vi "Polls.Compile.vi"(8 "error in (no error)":errorcluster, 11 "Section Ref in":T6 format="%.0x") -> (0 "error out":errorcluster, 1 "Poll Settings":T1[](array[typedef]), 2 "Service Channels":T3[](array[typedef]) {"Signal.Cmd.Refs"."Signal Refs" format="%.0x"; "Signal.Cmd.Info"."Signals"."Byte Order" items=["Little Endian", "Big Endian"]; "Signal.Cmd.Info"."Signals"."Data Type" items=["Signed", "Unsigned", "IEEE Float"]; "Settings.Refs"."Signal Refs" format="%.0x"; "Signal.Resp.Refs"."Signal Refs" format="%.0x"; "Signal.Resp.Info"."Signals"."Byte Order" items=["Little Endian", "Big Endian"]; "Signal.Resp.Info"."Signals"."Data Type" items=["Signed", "Unsigned", "IEEE Float"]; "Trigger.Refs"."Signal Refs" format="%.0x"; "Status.Refs"."Signal Refs" format="%.0x"}, 3 "Section Ref out":T6 format="%.0x")   [LabVIEW 2019, in "Diagnostics Addon System Explorer.lvlib"]
uses:
  Diagnostics Addon System Explorer.lvlib
  <vilib>/NI VeriStand/Custom Device API/Custom Device Item Ref.ctl
  Types/Service.Export.ctl
  Types/Frame.Ref.ctl
  Addon Shared/Types/Type.ctl
  Addon Shared/Types/Frame.Compile.ctl
  Addon Shared/Types/Signal.ctl
  Addon Shared/Types/Poll.Compiled.ctl
  Addon Shared/Types/DPID.Rate.ctl
  Types/FG.Action.ctl
  Addon Shared/SubVIs/Constants.vi
  <vilib>/NI VeriStand/Custom Device Tools/Custom Device Utility Library/NI VeriStand - Search for All Items by GUID.vi
  <vilib>/NI VeriStand/Custom Device Tools/Custom Device Utility Library/NI VeriStand - Search for Item by GUID.vi
  <vilib>/NI VeriStand/Custom Device API/NI VeriStand - Get Item Children.vi
  <vilib>/NI VeriStand/Custom Device Tools/Custom Device Utility Library/NI VeriStand - Search for Item by Name.vi
  <vilib>/NI/NI VeriStand Advanced SysDef API/SysDef API/SysDef.Property.Set.vi
  <vilib>/NI/NI VeriStand Advanced SysDef API/_SubVIs/SysDef.Property.Set.U32.vi
  <vilib>/NI VeriStand/Custom Device API/NI VeriStand - Get Item Property.vi
  <vilib>/NI VeriStand/Custom Device API/Get Item Property (U32).vi
  <vilib>/NI VeriStand/Custom Device Tools/Custom Device Utility Library/Custom Device Utility Library.lvlib
  <vilib>/NI VeriStand/Custom Device API/Custom Device API.lvlib
  Addon Shared/Diagnostics Addon Shared.lvlib
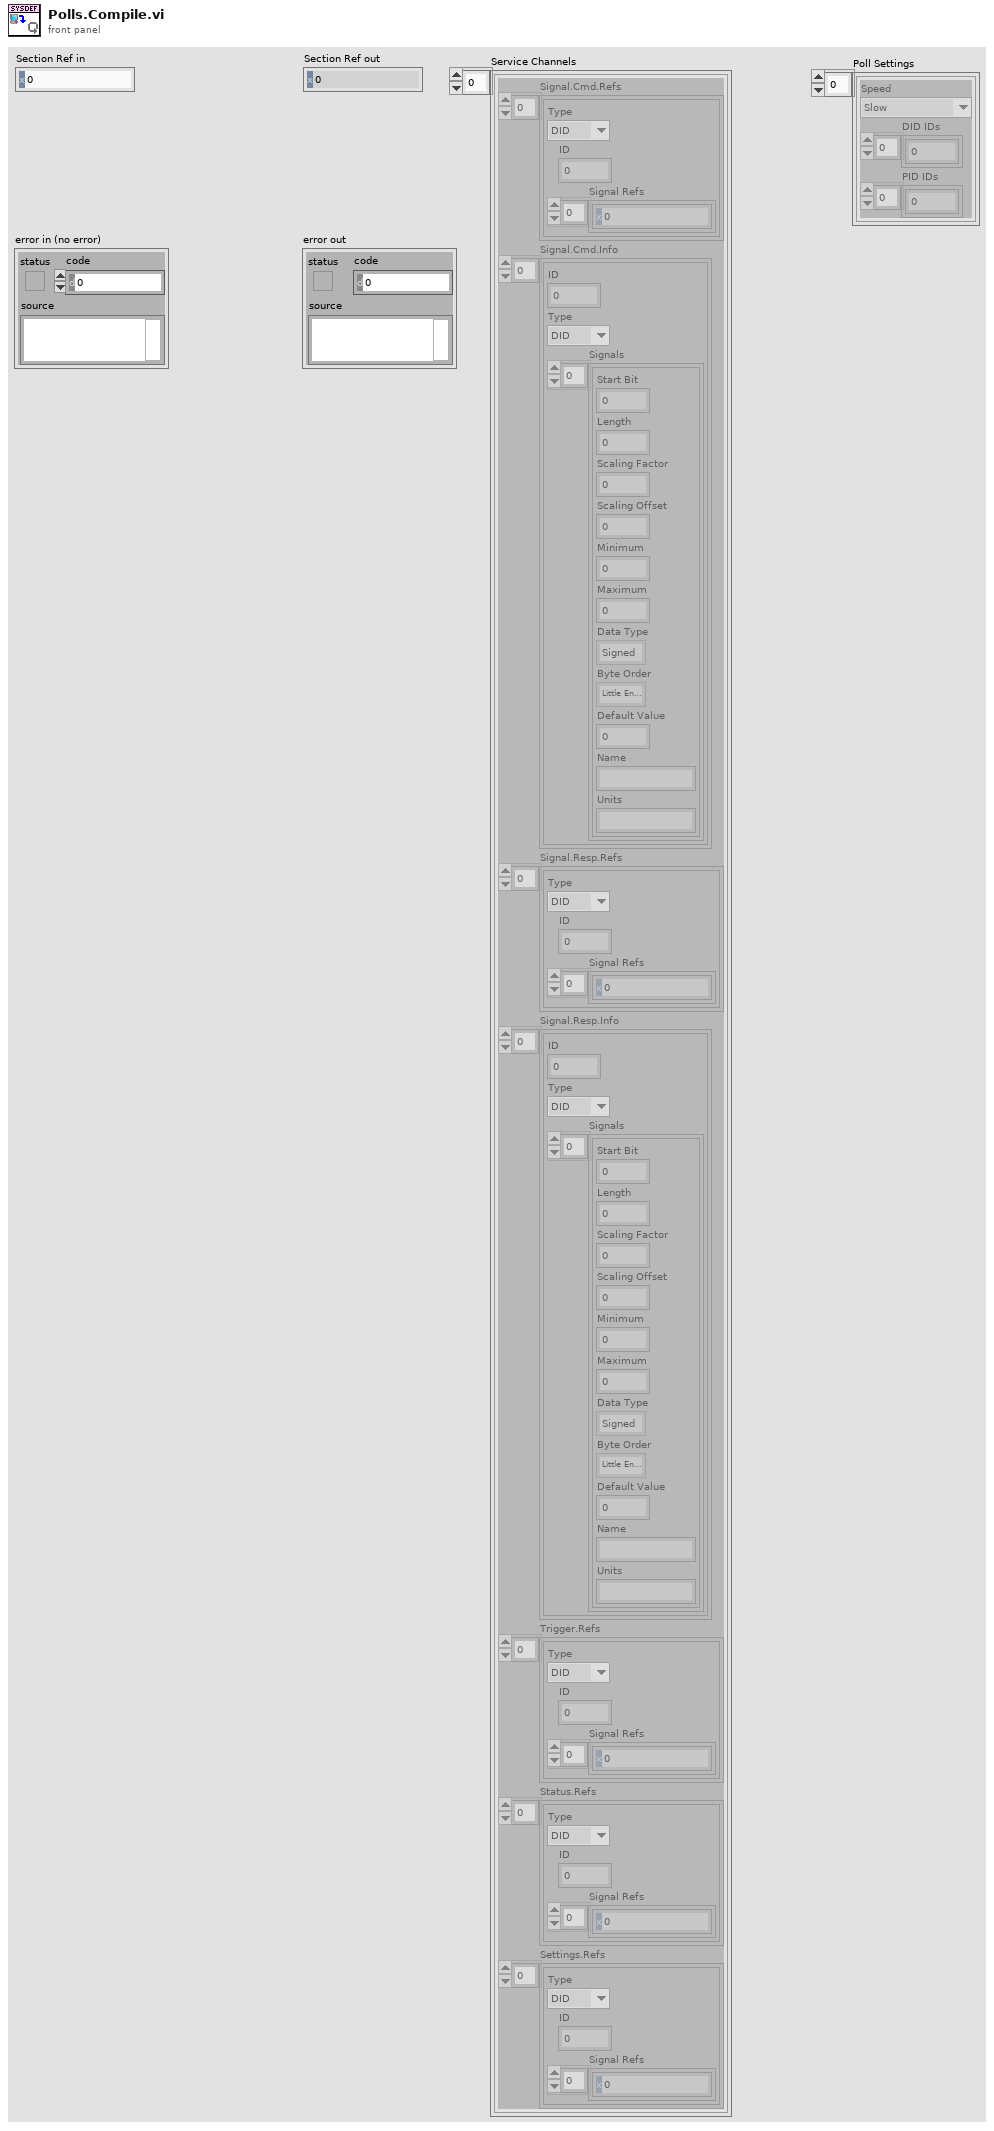
[diagram p1: front panel]
types:
  T1 = typedef "Diagnostics Addon Shared.lvlib/Poll.Compiled.ctl" = cluster{"Speed":T2, "DID IDs":u32[], "PID IDs":u32[]}
  T2 = typedef "Diagnostics Addon Shared.lvlib/DPID.Rate.ctl" = enum16{"Slow", "Medium", "Fast"}
  T3 = typedef "Diagnostics Addon System Explorer.lvlib/Service.Export.ctl" = cluster{"Signal.Cmd.Refs":T4[], "Signal.Cmd.Info":T7[], "Signal.Resp.Refs":T4[], "Signal.Resp.Info":T7[], "Trigger.Refs":T4[], "Status.Refs":T4[], "Settings.Refs":T4[]}
  T4 = typedef "Diagnostics Addon System Explorer.lvlib/Frame.Ref.ctl" = cluster{"Type":T5, "ID":u32, "Signal Refs":T6[]}
  T5 = typedef "Diagnostics Addon Shared.lvlib/Type.ctl" = enum16{"DID", "CDID", "PID", "CPID", "Read Memory", "Write Memory", "IO Control", "Routine Start", "Routine Request", "Routine Stop", "User Defined", "DTC Control", "Clear DTCs", "Read DTCs", "Start DTCs", "DTC Change Count", "Tester Present", "Unlock ECU", "Reset ECU", "Diag Session Control", "Communication Control", "DPID Control", "Poll Control", "Diag CAN Control"}
  T6 = typedef "Custom Device API.lvlib/Custom Device Item Ref.ctl" = u64
  T7 = typedef "Diagnostics Addon Shared.lvlib/Frame.Compile.ctl" = cluster{"ID":u32, "Type":T5, "Signals":T8[]}
  T8 = typedef "Diagnostics Addon Shared.lvlib/Signal.ctl" = cluster{"Start Bit":u32, "Length":u32, "Scaling Factor":dbl, "Scaling Offset":dbl, "Minimum":dbl, "Maximum":dbl, "Data Type":u32, "Byte Order":u32, "Default Value":dbl, "Name":string, "Units":string}
  T9 = typedef "Diagnostics Addon System Explorer.lvlib/FG.Action.ctl" = enum16{"Get", "Set"}
  T10 = typedef "Diagnostics Addon System Explorer.lvlib/Poll.Settings.ctl" = cluster{"Input Channels":T11[], "Speed":T2}
  T11 = typedef "Diagnostics Addon System Explorer.lvlib/Poll.LinkedNode.ctl" = cluster{"Node ID":u64}
  T12 = typedef "Custom Device API.lvlib/Custom Device Item Info.ctl" = cluster{"Name":string, "Is Channel":bool, "GUID":string, "Is Waveform":bool}
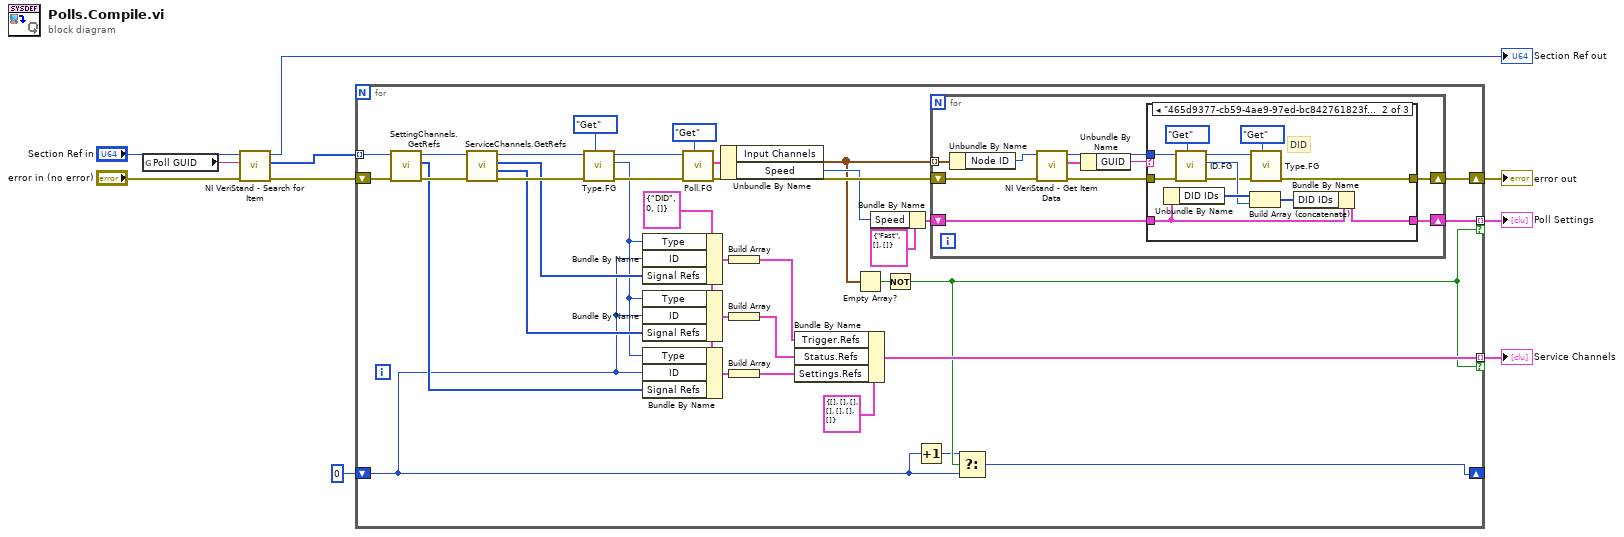
[diagram p0: block diagram]
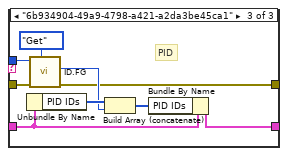
[diagram p3: hidden frame]
diagram:
  n1 = global read "Constants.vi" "Poll GUID"() -> (w10:string)
  n2 = call-poly <vilib>:"NI VeriStand - Search for Item.vi"("error in"="error in (no error)", "Item GUID"=w10, "Section Ref in"="Section Ref in") -> ("error out"=w9:errorcluster, "Item Refs"=w8:T6[], "Section Ref out"=→"Section Ref out":T6)  [unwired: 5 in, 1 out]
  n3 = for {
    tunnel: w8 -> [w15] mode=indexing
    shift-right: [w40] -> w5
    shift-left: w9 -> [w38]
    tunnel: [w41] -> w2 mode=indexing if=w14
    tunnel: [w17] -> w3 mode=indexing if=w14
    shift-right: [w13] -> _
    shift-left: 0 -> [w11]
    w27 = T4 {"Type"=enum."DID", "ID"=0, "Signal Refs"=[]} ("cluster")
    n4 = call "SettingChannels.GetRefs.vi"("error in (no error)"=w38, "Item Ref in"=w15) -> ("error out"=w34:errorcluster, "Settings"=w24:T6[], "Section Ref out"=w33:T6)  [unwired: 7 in]
    n5 = call "ServiceChannels.GetRefs.vi"("error in (no error)"=w34, "Item Ref in"=w33) -> ("error out"=w32:errorcluster, "Status"=w25:T6[], "Trigger"=w26:T6[], "Section Ref out"=w31:T6)  [unwired: 6 in]
    n6 = call "Type.FG.vi"("Action"=FG.Action."Get", "error in (no error)"=w32, "Device Item Ref in"=w31) -> ("error out"=w37:errorcluster, "Type"=w20:T5, "Device Item Ref out"=w16:T6)  [unwired: 6 in]
    n7 = Bundle By Name(cluster=w27, "Type"=w20, "ID"=w11, "Signal Refs"=w26) -> (w30:T4)
    n8 = Bundle By Name(cluster=w27, "Type"=w20, "ID"=w11, "Signal Refs"=w25) -> (w29:T4)
    n9 = Bundle By Name(cluster=w27, "Type"=w20, "ID"=w11, "Signal Refs"=w24) -> (w28:T4)
    n10 = call "Poll.FG.vi"("Action"=FG.Action."Get", "error in"=w37, "Parent Ref"=w16) -> ("error out"=w43:errorcluster, "Selected Channels out"=w44:T10)  [unwired: 6 in, 1 out]
    n11 = Unbundle By Name(w44) -> ("Input Channels"=w19:T11[], "Speed"=w39:T2)
    n12 = Build Array(w30) -> (w23:T4[])
    n13 = Build Array(w29) -> (w22:T4[])
    n14 = Build Array(w28) -> (w21:T4[])
    n15 = Bundle By Name(cluster=T3 {"Signal.Cmd.Refs"=[], "Signal.Cmd.Info"=[], "Signal.Resp.Refs"=[], "Signal.Resp.Info"=[], "Trigger.Refs"=[], "Status.Refs"=[], "Settings.Refs"=[]}, "Trigger.Refs"=w23, "Status.Refs"=w22, "Settings.Refs"=w21) -> (w17:T3)
    n16 = Empty Array?(array=w19) -> (empty?=w18:bool)
    n17 = Bundle By Name(cluster=T1 {"Speed"=enum."Fast", "DID IDs"=[], "PID IDs"=[]}, "Speed"=w39) -> (w42:T1)
    n18 = Not(x=w18) -> (.not. x?=w14:bool)
    n19 = Increment(x=w11) -> (x+1=w12:i32)
    n20 = for {
      tunnel: w19 -> [w56] mode=indexing
      shift-right: [w49] -> w40
      shift-left: w43 -> [w54]
      shift-right: [w48] -> w41
      shift-left: w42 -> [w50]
      n21 = Unbundle By Name(w56) -> ("Node ID"=w53:u64)
      n22 = call <vilib>:"NI VeriStand - Get Item Data.vi"("error in (no error)"=w54, "Item Ref in"=w53) -> ("error out"=w51:errorcluster, "Item Info"=w55:T12, "Item Ref out"=w47:T6)  [unwired: 6 in, 1 out]
      n23 = Unbundle By Name(w55) -> ("GUID"=w52:string)
      n24 = case shown="\"465d9377-cb59-4ae9-97ed-bc842761823f\"" w52 {
        tunnel: w51 -> [w58 w69 w78]
        tunnel: w50 -> [w57 w68 w75]
        tunnel: [w58 w60 w72] -> w49
        tunnel: [w57 w63 w71] -> w48
        tunnel: w47 -> [_ w65 w74]
        frame Default {
        }
        frame "465d9377-cb59-4ae9-97ed-bc842761823f" {
          # "DID"
          n25 = Unbundle By Name(w68) -> ("DID IDs"=w67:u32[])
          n26 = call "ID.FG.vi"("Action"=FG.Action."Get", "error in (no error)"=w69, "Device Item Ref in"=w65) -> ("error out"=w61:errorcluster, "ID"=w66:u32, "Device Item Ref out"=w59:T6)  [unwired: 6 in]
          n27 = Build Array (concatenate)(w67, w66) -> (w64:u32[])
          n28 = call "Type.FG.vi"("Action"=FG.Action."Get", "error in (no error)"=w61, "Device Item Ref in"=w59) -> ("error out"=w60:errorcluster)  [unwired: 6 in, 2 out]
          n29 = Bundle By Name(cluster=w68, "DID IDs"=w64) -> (w63:T1)
        }
        frame "6b934904-49a9-4798-a421-a2da3be45ca1" {
          # "PID"
          n30 = Unbundle By Name(w75) -> ("PID IDs"=w77:u32[])
          n31 = call "ID.FG.vi"("Action"=FG.Action."Get", "error in (no error)"=w78, "Device Item Ref in"=w74) -> ("error out"=w72:errorcluster, "ID"=w73:u32)  [unwired: 6 in, 1 out]
          n32 = Build Array (concatenate)(w77, w73) -> (w76:u32[])
          n33 = Bundle By Name(cluster=w75, "PID IDs"=w76) -> (w71:T1)
        }
      }
    }
    n34 = Select(t=w12, s=w14, f=w11) -> (s? t:f=w13:i32)
  }
  "error out" <- w5
  "Service Channels" <- w3
  "Poll Settings" <- w2
